vi "Refactor Object for File Rename.vi"(8 "error in (no error)":errorcluster, 10 "renamed files":T1[](array[typedef]), 11 "object reference in":refnum<vi>) -> (0 "error out":errorcluster, 1 "refactored dependency":bool, 2 "refactor result":T2, 3 "object reference out":refnum<vi>)   [LabVIEW 2021, in "MeasurementService Editor.lvlib"]
uses:
  MeasurementService Editor.lvlib
  Refactor Object Result.ctl
  Rename Refactor Mapping Info.ctl
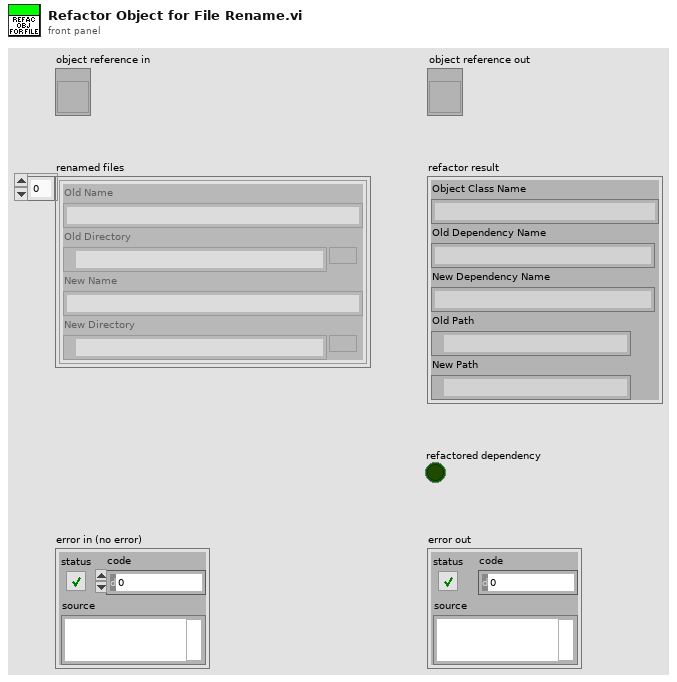
[diagram p1: front panel]
types:
  T1 = typedef "MeasurementService Editor.lvlib/Rename Refactor Mapping Info.ctl" = cluster{"Old Name":string, "Old Directory":path, "New Name":string, "New Directory":path}
  T2 = typedef "MeasurementService Editor.lvlib/Refactor Object Result.ctl" = cluster{"Object Class Name":string, "Old Dependency Name":string, "New Dependency Name":string, "Old Path":path, "New Path":path}
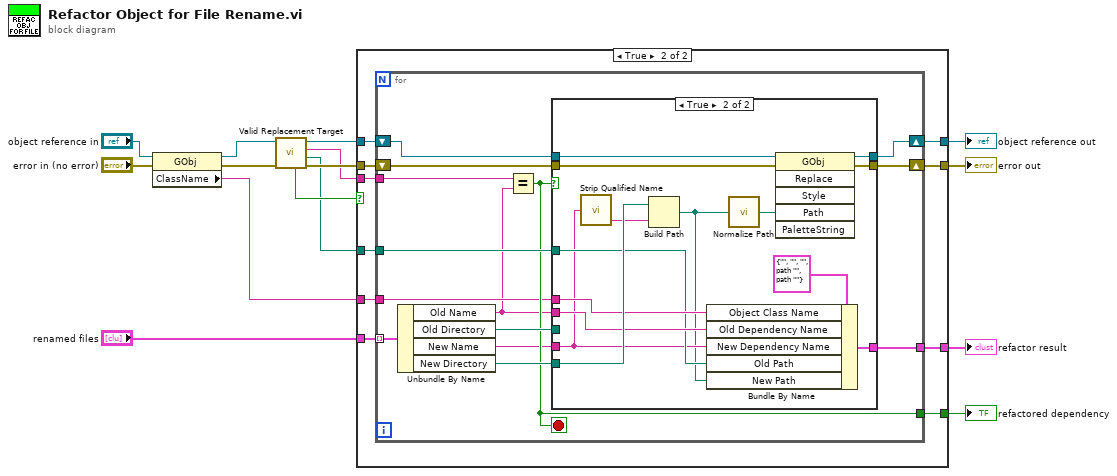
[diagram p0: block diagram]
diagram:
  n1 = property class="GObj"(reference="object reference in", error in="error in (no error)") -> (reference out=w2:refnum<vi>, error out=w8:errorcluster, "ClassName"=w12:string)
  n2 = call "Valid Replacement Target.vi"("error in (no error)"=w8, "object reference in"=w2) -> ("error out"=w7:errorcluster, "missing path"=w4:path, "missing name"=w3:string, "object reference out"=w1:refnum<vi>, "valid replacement target"=w5:bool)  [unwired: 5 in]
  n3 = case shown="True" w5 {
    tunnel: w1 -> [w16 w27]
    tunnel: w7 -> [w17 w26]
    tunnel: w3 -> [_ w24]
    tunnel: [w17 w20] -> w15
    tunnel: [w16 w21] -> w11
    tunnel: w12 -> [_ w22]
    tunnel: w4 -> [_ w23]
    tunnel: "renamed files" -> [_ w25]
    tunnel: [_ w19] -> w9
    tunnel: [_ w18] -> w10
    frame False {
    }
    frame True {
      n4 = for {
        shift-right: [w36] -> w20
        shift-left: w26 -> [w38]
        shift-right: [w37] -> w21
        shift-left: w27 -> [w39]
        tunnel: w25 -> [w41] mode=indexing
        tunnel: w24 -> [w40]
        tunnel: w23 -> [w34]
        tunnel: [w32] -> w19
        tunnel: w22 -> [w31]
        tunnel: [w28] -> w18
        stop <- w32 stop-if-true
        n5 = Unbundle By Name(w41) -> ("Old Name"=w30:string, "Old Directory"=w35:path, "New Name"=w29:string, "New Directory"=w33:path)
        n6 = Equal?(x=w40, y=w30) -> (x = y?=w32:bool)
        n7 = case shown="True" w32 {
          tunnel: w39 -> [w43 w54]
          tunnel: w38 -> [w42 w48]
          tunnel: [w43 w55] -> w37
          tunnel: [w42 w56] -> w36
          tunnel: w35 -> [_ _]
          tunnel: w34 -> [_ w50]
          tunnel: w33 -> [_ w57]
          tunnel: w31 -> [_ w52]
          tunnel: w30 -> [_ w51]
          tunnel: w29 -> [_ w47]
          tunnel: [_ w49] -> w28
          frame False {
          }
          frame True {
            n8 = call "Strip Qualified Name.vi"("name"=w47) -> ("last name"=w46:string)  [unwired: 5 in, 1 out]
            n9 = Build Path(base path=w57, name or relative path=w46) -> (appended path=w45:path)
            n10 = Bundle By Name(cluster=T2 {"Object Class Name"="", "Old Dependency Name"="", "New Dependency Name"="", "Old Path"=path "", "New Path"=path ""} ("Rename Refactor Result"), "Object Class Name"=w52, "Old Dependency Name"=w51, "New Dependency Name"=w47, "Old Path"=w50, "New Path"=w45) -> (w49:T2)
            n11 = call "Normalize Path.vi"("path"=w45) -> ("normalized path"=w44:path)
            n12 = invoke class="GObj" method="Replace"(reference=w54, error in=w48, "Path"=w44) -> (reference out=w55:refnum<vi>, error out=w56:errorcluster)  [unwired: 3 in, 4 out]
          }
        }
      }
    }
  }
  "error out" <- w15
  "object reference out" <- w11
  "refactor result" <- w10
  "refactored dependency" <- w9
